vi "Copy .LLB to NI VeriStand dir.vi"(5 "Files Generated by Build":path[](array[path]), 6 "Top Level/Always Included VIs":path[](array[path]), 7 "Destination Path":path, 8 "error in (no error)":errorcluster, 9 "Target Name":string, 10 "Build Specification Name":string, 11 "Project Path":path) -> (0 "error out":errorcluster)   [LabVIEW 2020]
doc: "This VI is called after each run of a build specification. The VI will copy the generated LLB (Engine or System Explorer) into the VeriStand Custom Device folder (...\\Documents\\National Instruments\\NI VeriStand 2013...)."
uses:
  C:/Users/ppathak/Downloads/NationalInstruments.VeriStand.dll
  Users/ppathak/Downloads/NationalInstruments.VeriStand.dll
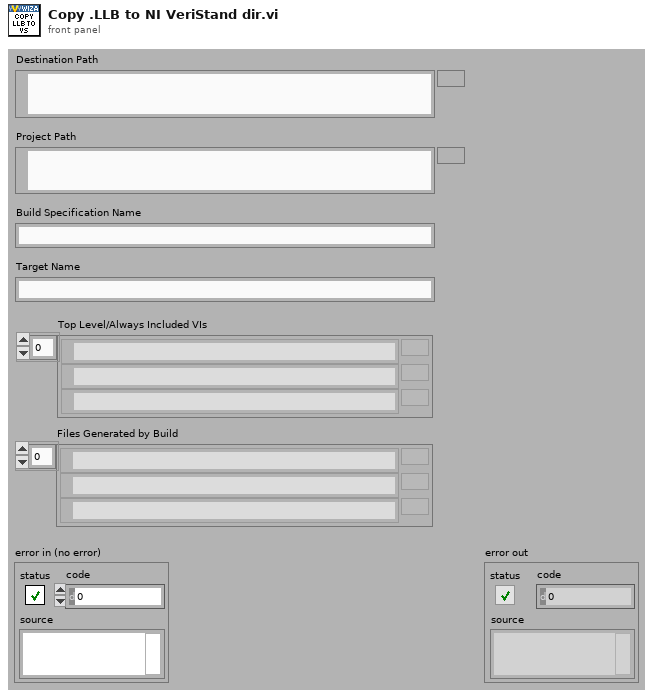
[diagram p1: front panel]
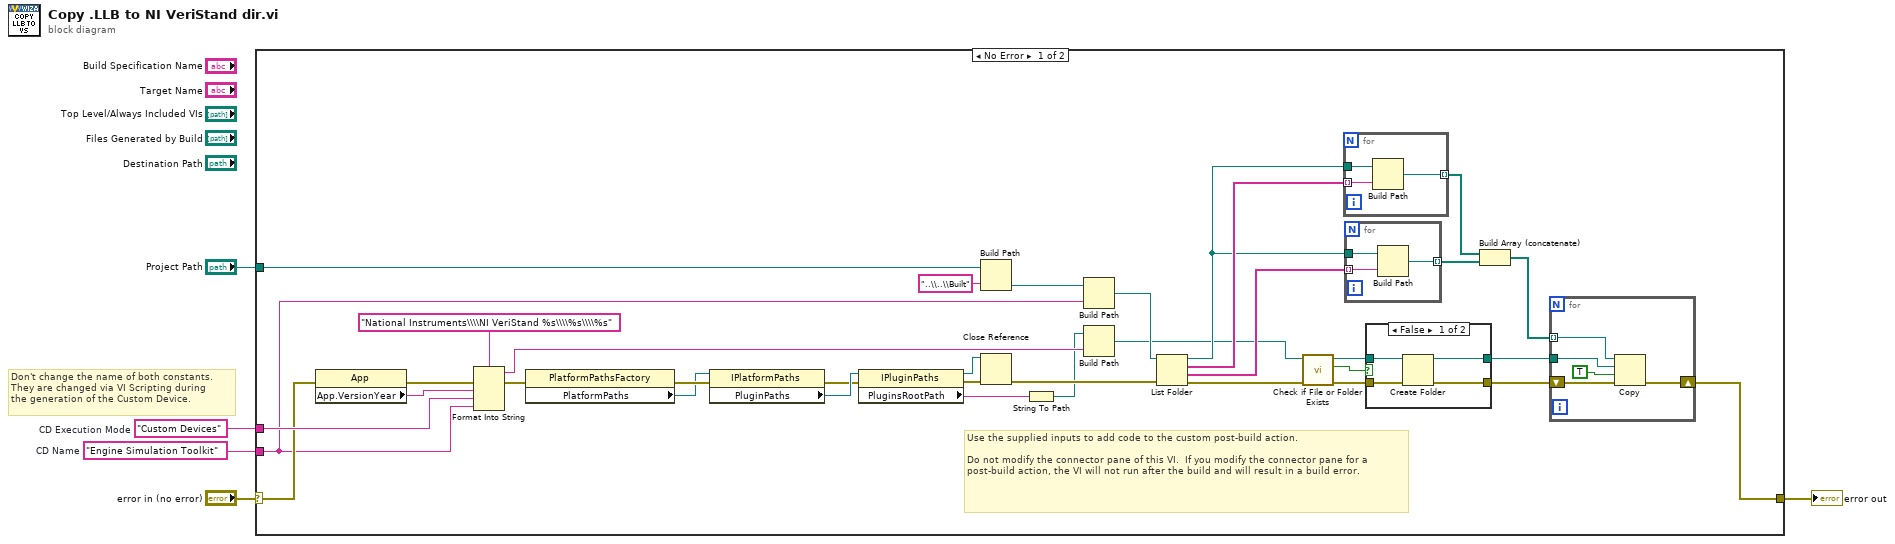
[diagram p0: block diagram]
diagram:
  w2 = "Engine Simulation Toolkit"  # CD Name
  w3 = "Custom Devices"  # CD Execution Mode
  # "Don't change the name of both constants.\nThey are changed via VI Scripting during\nthe generation of the Custom Device."
  n1 = case shown="No Error" "error in (no error)" {
    selector: "error in (no error)" -> [w21 w58]
    tunnel: [w24 w58] -> w1
    tunnel: "Project Path" -> [w18 _]
    tunnel: w3 -> [w22 _]
    tunnel: w2 -> [w20 _]
    frame No Error {
      # "Use the supplied inputs to add code to the custom post-build action.\n\nDo not modify the connector pane of this VI.  If you modify the connector pane for a post-build action, the VI will not run after the build and will result in a build error."
      n2 = property class="App"(error in=w21) -> (error out=w27:errorcluster, "App.VersionYear"=w26:string)  [unwired: 1 in, 1 out]
      n3 = Format Into String(format string="National Instruments\\\\NI VeriStand %s\\\\%s\\\\%s" ("name or relative path"), error in=w27, w26, w22, w20) -> (resulting string=w28:string, error out=w6:errorcluster)  [unwired: 1 in]
      n4 = property class="PlatformPathsFactory"(error in=w6) -> (error out=w14:errorcluster, "PlatformPaths"=w12:refnum<k24>)  [unwired: 1 in, 1 out]
      n5 = property class="IPlatformPaths"(reference=w12, error in=w14) -> (error out=w13:errorcluster, "PluginPaths"=w15:refnum<k24>)  [unwired: 1 out]
      n6 = property class="IPluginPaths"(reference=w15, error in=w13) -> (reference out=w9:refnum<k24>, error out=w10:errorcluster, "PluginsRootPath"=w11:string)
      n7 = Build Path(base path=w18, name or relative path="..\\..\\Built") -> (appended path=w29:path)
      n8 = Close Reference(reference=w9, error in (no error)=w10) -> (error out=w8:errorcluster)
      n9 = String To Path(string=w11) -> (path=w7:path)
      n10 = Build Path(base path=w29, name or relative path=w20) -> (appended path=w31:path)
      n11 = Build Path(base path=w7, name or relative path=w28) -> (appended path=w23:path)
      n12 = List Folder(path=w31, error in=w8) -> (path out=w33:path, filenames=w40:string[], folder names=w34:string[], error out=w30:errorcluster)  [unwired: 2 in]
      n13 = call <vilib>:"Check if File or Folder Exists.vi"("error in (no error)"=w30, "path"=w23) -> ("error out"=w35:errorcluster, "file or folder exists?"=w37:bool, "dup path"=w36:path)  [unwired: 7 in]
      n14 = for {
        tunnel: w40 -> [w56] mode=indexing
        tunnel: w33 -> [w57]
        tunnel: [w55] -> w39 mode=indexing
        n15 = Build Path(base path=w57, name or relative path=w56) -> (appended path=w55:path)
      }
      n16 = for {
        tunnel: w34 -> [w53] mode=indexing
        tunnel: w33 -> [w54]
        tunnel: [w52] -> w32 mode=indexing
        n17 = Build Path(base path=w54, name or relative path=w53) -> (appended path=w52:path)
      }
      n18 = case shown="False" w37 {
        tunnel: w36 -> [w44 w46]
        tunnel: w35 -> [w43 w45]
        tunnel: [w42 w46] -> w17
        tunnel: [w41 w45] -> w16
        frame False {
          n19 = Create Folder(path (use dialog)=w44, error in=w43) -> (created path=w42:path, error out=w41:errorcluster)  [unwired: 1 in, 1 out]
        }
        frame True {
        }
      }
      n20 = Build Array (concatenate)(w39, w32) -> (w38:path[])
      n21 = for {
        tunnel: w38 -> [w48] mode=indexing
        shift-right: [w49] -> w24
        shift-left: w16 -> [w50]
        tunnel: w17 -> [w47]
        n22 = Copy(8:w50, 9:TRUE ("overwrite (F)"), 10:w47, 11:w48) -> (0:w49:errorcluster)  [unwired: 1 in, 2 out]
      }
    }
    frame Error {
    }
  }
  "error out" <- w1
